vi "Purge.vi"(5 "Digital I/O Pin":u8=7, 7 "Arduino Resource":T1={"VISA resource"="GlueCTRL", "Board Type"=enum."Uno", "Connection Type"=enum."USB / Serial", "Bytes Per Packet (15)"=15}, 9 "Axis Speeds":T3={"X [mm/s]"=25.0, "Y [mm/s]"=25.0, "Z [mm/s]"=10.0}, 10 "Start Position [mm]":dbl[](array[numeric]), 11 ".NET Refnum In":refnum<k24>) -> ()   [LabVIEW 2016]
uses:
  C:/Users/Aerotech/Documents/BNLStaveAssembly-blueprint/Bin/Aerotech.A3200.dll
  BNLStaveAssembly-blueprint/Bin/Aerotech.A3200.dll
  <vilib>/LabVIEW Interface for Arduino/Type Defs/Arduino Resource.ctl
  <vilib>/LabVIEW Interface for Arduino/Type Defs/Board Type.ctl
  <vilib>/LabVIEW Interface for Arduino/LabVIEW Interface for Arduino.lvlib
panel:
  in  "Absolute Purge Height [mm]":dbl=-30.0 format="%#_13g"
  in  "Relative Change in X, Y to Purge [mm]":dbl[](array[numeric])=[0.0, -150.0, 0.0]
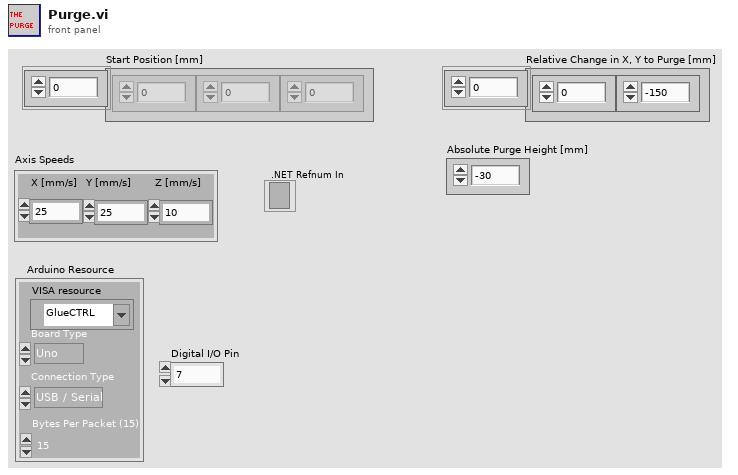
[diagram p1: front panel]
types:
  T1 = typedef "LabVIEW Interface for Arduino.lvlib/Arduino Resource.ctl" = cluster{"VISA resource":refnum<visa-resource-name>, "Board Type":T2, "Connection Type":enum8{"USB / Serial"}, "Bytes Per Packet (15)":u8}
  T2 = typedef "LabVIEW Interface for Arduino.lvlib/Board Type.ctl" = enum16{"Uno", "Dimuelanove w/Atmega 328", "Mega 2560"}
  T3 = cluster{"X [mm/s]":dbl, "Y [mm/s]":dbl, "Z [mm/s]":dbl}
  T4 = cluster{"Start Position [mm][0]":dbl, "Start Position [mm][1]":dbl, "Start Position [mm][2]":dbl}
  T5 = cluster{"Final X":dbl, "Final Y":dbl, "Final Z":dbl}
  T6 = cluster{"Final Position[0]":dbl, "Final Position[1]":dbl, "Final Position[2]":dbl}
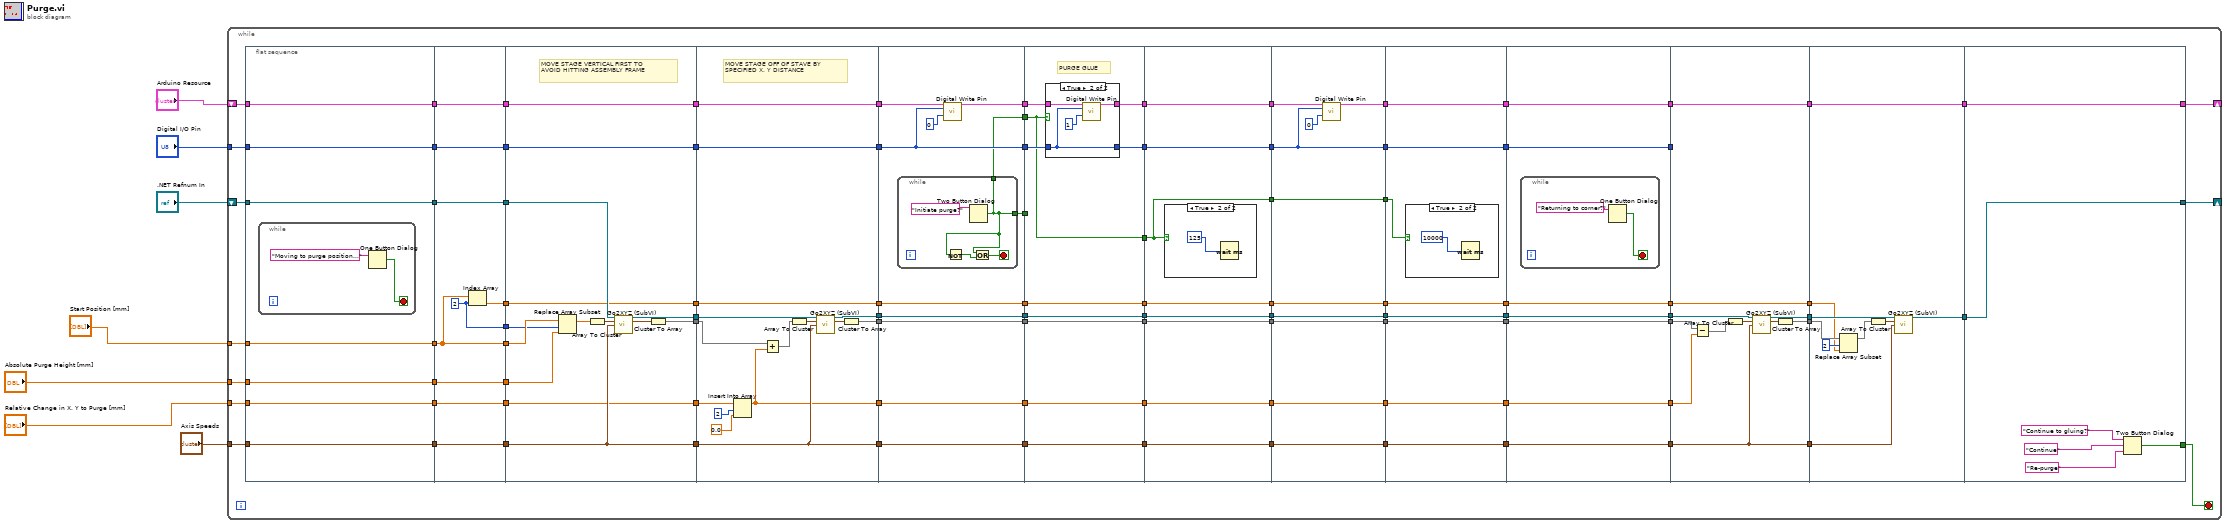
[diagram p0: block diagram]
diagram:
  n1 = while {
    tunnel: "Start Position [mm]" -> [w100]
    tunnel: "Relative Change in X, Y to Purge [mm]" -> [w99]
    tunnel: "Axis Speeds" -> [w98]
    shift-right: [w94] -> _
    shift-left: ".NET Refnum In" -> [w97]
    tunnel: "Digital I/O Pin" -> [w92]
    shift-right: [w87] -> _
    shift-left: "Arduino Resource" -> [w93]
    tunnel: "Absolute Purge Height [mm]" -> [w68]
    stop <- w101 stop-if-true
    n2 = flat-sequence {
      tunnel: [w108] -> w47
      tunnel: w100 -> [w108]
      tunnel: w99 -> [w107]
      tunnel: [w107] -> w45
      tunnel: [w106] -> w43
      tunnel: w98 -> [w106]
      tunnel: [w105] -> w41
      tunnel: w97 -> [w105]
      tunnel: [w104] -> w39
      tunnel: w93 -> [w104]
      tunnel: w92 -> [w103]
      tunnel: [w103] -> w37
      tunnel: w68 -> [w102]
      tunnel: [w102] -> w35
      tunnel: w47 -> [w113]
      tunnel: [w113] -> w46
      tunnel: w45 -> [w119]
      tunnel: [w119] -> w44
      tunnel: w43 -> [w118]
      tunnel: [w118] -> w42
      tunnel: w41 -> [w117]
      tunnel: [w117] -> w40
      tunnel: w39 -> [w116]
      tunnel: [w116] -> w38
      tunnel: w37 -> [w115]
      tunnel: [w115] -> w36
      tunnel: w35 -> [w114]
      tunnel: [w114] -> w34
      tunnel: [w112] -> w33
      tunnel: [w111] -> w32
      tunnel: w46 -> [w122]
      tunnel: w44 -> [w126]
      tunnel: w42 -> [w131]
      tunnel: w40 -> [w133]
      tunnel: [w132] -> w78
      tunnel: [w131] -> w76
      tunnel: w38 -> [w130]
      tunnel: [w130] -> w74
      tunnel: w36 -> [w129]
      tunnel: [w129] -> w72
      tunnel: [w127] -> w70
      tunnel: [w126] -> w69
      tunnel: w34 -> [w124]
      tunnel: [w121] -> w53
      tunnel: w33 -> [w121]
      tunnel: w32 -> [w120]
      tunnel: w78 -> [w146]
      tunnel: [w145] -> w77
      tunnel: w76 -> [w138]
      tunnel: [w138] -> w75
      tunnel: w74 -> [w148]
      tunnel: [w148] -> w73
      tunnel: w72 -> [w147]
      tunnel: [w147] -> w71
      tunnel: w70 -> [w143]
      tunnel: w69 -> [w139]
      tunnel: [w136] -> w67
      tunnel: [w135] -> w56
      tunnel: w53 -> [w134]
      tunnel: [w134] -> w52
      tunnel: [w159] -> w91
      tunnel: w77 -> [w159]
      tunnel: [w158] -> w90
      tunnel: w75 -> [w158]
      tunnel: w73 -> [w156]
      tunnel: w71 -> [w154]
      tunnel: [w155] -> w89
      tunnel: [w154] -> w86
      tunnel: [w153] -> w84
      tunnel: [w152] -> w83
      tunnel: w67 -> [w151]
      tunnel: [w151] -> w60
      tunnel: [w150] -> w57
      tunnel: w56 -> [w150]
      tunnel: w52 -> [w149]
      tunnel: [w149] -> w48
      tunnel: w91 -> [w173]
      tunnel: [w173] -> w82
      tunnel: w90 -> [w172]
      tunnel: [w172] -> w81
      tunnel: w89 -> [w171]
      tunnel: [w170] -> w80
      tunnel: [w168] -> w79
      tunnel: w86 -> [w169]
      tunnel: w84 -> [w164]
      tunnel: w83 -> [_]
      tunnel: [w167] -> w61
      tunnel: w60 -> [w167]
      tunnel: [w166] -> w58
      tunnel: w57 -> [w166]
      tunnel: [w165] -> w49
      tunnel: w48 -> [w165]
      tunnel: [w164] -> w31
      tunnel: w82 -> [w187]
      tunnel: [w187] -> w30
      tunnel: w81 -> [w186]
      tunnel: [w186] -> w29
      tunnel: w80 -> [w185]
      tunnel: [w185] -> w28
      tunnel: w79 -> [w184]
      tunnel: [w184] -> w27
      tunnel: [w183] -> w26
      tunnel: w61 -> [w183]
      tunnel: [w182] -> w25
      tunnel: w58 -> [w182]
      tunnel: [w181] -> w24
      tunnel: w49 -> [w181]
      tunnel: w31 -> [w180]
      tunnel: [w180] -> w8
      tunnel: w30 -> [w198]
      tunnel: [w198] -> w23
      tunnel: w29 -> [w197]
      tunnel: [w197] -> w21
      tunnel: w28 -> [w193]
      tunnel: [w192] -> w19
      tunnel: w27 -> [w190]
      tunnel: [w190] -> w17
      tunnel: w26 -> [w196]
      tunnel: [w196] -> w15
      tunnel: w25 -> [w195]
      tunnel: [w195] -> w13
      tunnel: w24 -> [w194]
      tunnel: [w194] -> w11
      tunnel: [w189] -> w9
      tunnel: w8 -> [w189]
      tunnel: w23 -> [w206]
      tunnel: [w206] -> w22
      tunnel: w21 -> [w205]
      tunnel: [w205] -> w20
      tunnel: w19 -> [w204]
      tunnel: [w204] -> w18
      tunnel: w17 -> [w203]
      tunnel: [w203] -> w16
      tunnel: w15 -> [w202]
      tunnel: [w202] -> w14
      tunnel: w13 -> [w201]
      tunnel: [w201] -> w12
      tunnel: w11 -> [w200]
      tunnel: [w200] -> w10
      tunnel: w9 -> [w199]
      tunnel: w22 -> [w214]
      tunnel: [w214] -> w96
      tunnel: w20 -> [w213]
      tunnel: [w213] -> w95
      tunnel: w18 -> [w208]
      tunnel: [w208] -> w88
      tunnel: w16 -> [w212]
      tunnel: [w212] -> w85
      tunnel: [w211] -> w62
      tunnel: w14 -> [w211]
      tunnel: [w210] -> w59
      tunnel: w12 -> [w210]
      tunnel: [w209] -> w50
      tunnel: w10 -> [w209]
      tunnel: w96 -> [w226]
      tunnel: w95 -> [w218]
      tunnel: [w225] -> w66
      tunnel: [w224] -> w64
      tunnel: w88 -> [w224]
      tunnel: w85 -> [_]
      tunnel: w62 -> [w223]
      tunnel: w59 -> [w221]
      tunnel: [w219] -> w55
      tunnel: [w218] -> w54
      tunnel: [w217] -> w51
      tunnel: w50 -> [w217]
      tunnel: w66 -> [w235]
      tunnel: [w234] -> w65
      tunnel: w64 -> [w236]
      tunnel: [w236] -> w63
      tunnel: w55 -> [w231]
      tunnel: w54 -> [w232]
      tunnel: w51 -> [w229]
      tunnel: [w241] -> w101
      tunnel: w65 -> [w240]
      tunnel: [w240] -> w94
      tunnel: [w239] -> w87
      tunnel: w63 -> [w239]
      frame #0 {
        n3 = while {
          stop <- w109 stop-if-true
          n4 = One Button Dialog(message="Moving to purge position...") -> (true=w109:bool)  [unwired: 1 in]
        }
      }
      frame #1 {
        w111 = 2 ("index")
        n5 = Index Array(array=w113, index=w111) -> (element=w112:dbl)
      }
      frame #2 {
        # "MOVE STAGE VERTICAL FIRST TO\nAVOID HITTING ASSEMBLY FRAME"
        n6 = Replace Array Subset(array=w122, new element=w124, index=w120) -> (w123:dbl[])
        n7 = Array To Cluster(array=w123) -> (cluster=w125:T4)
        n8 = call "Go2XYZ (SubVI).vi"(".NET Refnum in"=w133, "Go to Coordinates"=w125, "Axis Speeds"=w131) -> (".NET Refnum out"=w132:refnum<k24>, "Final Position"=w128:T5)  [unwired: 8 in, 3 out]
        n9 = Cluster To Array(cluster=w128) -> (array=w127:dbl[])
      }
      frame #3 {
        # "MOVE STAGE OFF OF STAVE BY\nSPECIFIED X, Y DISTANCE"
        n10 = Insert Into Array(array=w139, index=2, new element=0.0 ("new element/subarray")) -> (w135:dbl[])
        n11 = Add(x=w143, y=w135) -> (x+y=w142:dbl[])
        n12 = Array To Cluster(array=w142) -> (cluster=w144:cluster{"[0]":dbl, "[1]":dbl, "[2]":dbl})
        n13 = call "Go2XYZ (SubVI).vi"(".NET Refnum in"=w146, "Go to Coordinates"=w144, "Axis Speeds"=w138) -> (".NET Refnum out"=w145:refnum<k24>, "Final Position"=w137:T5)  [unwired: 8 in, 3 out]
        n14 = Cluster To Array(cluster=w137) -> (array=w136:dbl[])
      }
      frame #4 {
        n15 = while {
          tunnel: [w160] -> w153
          tunnel: [w160] -> w152
          stop <- w161 stop-if-true
          n16 = Two Button Dialog(message="Initiate purge?") -> (T button?=w160:bool)  [unwired: 2 in]
          n17 = Not(x=w160) -> (.not. x?=w162:bool)
          n18 = Or(x=w160, y=w162) -> (x .or. y?=w161:bool)
        }
        n19 = call <vilib>:"Digital Write Pin.vi"("Arduino Resource"=w156, "Digital I/O Pin (0)"=w154, "Value (0)"=u8 0) -> ("Arduino Resource"=w155:T1)  [unwired: 11 in, 1 out]
      }
      frame #5 {
        # "PURGE GLUE"
        n20 = case shown="True" w164 {
          tunnel: w171 -> [w174 w178]
          tunnel: [w174 w177] -> w170
          tunnel: w169 -> [w175 w176]
          tunnel: [w175 w176] -> w168
          frame False {
          }
          frame True {
            n21 = call <vilib>:"Digital Write Pin.vi"("Arduino Resource"=w178, "Digital I/O Pin (0)"=w176, "Value (0)"=u8 1) -> ("Arduino Resource"=w177:T1)  [unwired: 11 in, 1 out]
          }
        }
      }
      frame #6 {
        n22 = case shown="True" w180 {
          frame False {
          }
          frame True {
            n23 = Wait (ms)(milliseconds to wait=u32 125) -> ()  [unwired: 1 out]
          }
        }
      }
      frame #7 {
        n24 = call <vilib>:"Digital Write Pin.vi"("Arduino Resource"=w193, "Digital I/O Pin (0)"=w190, "Value (0)"=u8 0) -> ("Arduino Resource"=w192:T1)  [unwired: 11 in, 1 out]
      }
      frame #8 {
        n25 = case shown="True" w199 {
          frame False {
          }
          frame True {
            n26 = Wait (ms)(milliseconds to wait=u32 10000) -> ()  [unwired: 1 out]
          }
        }
      }
      frame #9 {
        n27 = while {
          stop <- w216 stop-if-true
          n28 = One Button Dialog(message="Returning to corner?") -> (true=w216:bool)  [unwired: 1 in]
        }
      }
      frame #10 {
        n29 = Subtract(x=w223, y=w221) -> (x-y=w222:dbl[])
        n30 = Array To Cluster(array=w222) -> (cluster=w227:cluster{"[0]":dbl, "[1]":dbl, "[2]":dbl})
        n31 = call "Go2XYZ (SubVI).vi"(".NET Refnum in"=w226, "Go to Coordinates"=w227, "Axis Speeds"=w218) -> (".NET Refnum out"=w225:refnum<k24>, "Final Position"=w220:T5)  [unwired: 8 in, 3 out]
        n32 = Cluster To Array(cluster=w220) -> (array=w219:dbl[])
      }
      frame #11 {
        n33 = Replace Array Subset(array=w231, new element=w229, index=2) -> (w228:dbl[])
        n34 = Array To Cluster(array=w228) -> (cluster=w233:T6)
        n35 = call "Go2XYZ (SubVI).vi"(".NET Refnum in"=w235, "Go to Coordinates"=w233, "Axis Speeds"=w232) -> (".NET Refnum out"=w234:refnum<k24>)  [unwired: 8 in, 4 out]
      }
      frame #12 {
        n36 = Two Button Dialog(message="Continue to gluing?", 1:"Re-purge" ("F button name (\"Cancel\")"), 2:"Continue" ("T button name (\"OK\")")) -> (T button?=w241:bool)
      }
    }
  }
